vi "tower Controller.vi"(8 "error in":errorcluster) -> ()   [LabVIEW 2017]
doc: "This VI executes continuously carrying out the current operation and responding to updates or new operations. It will often contain the timing or control code that is difficult to place directly in TeleOp. This VI generally opens all sensors and motors and isolates the rest of the robot code from knowing how the operations are carried out."
uses:
  <vilib>/Rock Robotics/WPI/Framework/Completion Status.ctl
  tower Setpoints.ctl
  tower Operations.ctl
  <vilib>/Rock Robotics/SystemInterfaces/DIO/FPGA_DIOChannel.ctl
  <vilib>/Rock Robotics/WPI/Encoder/WPI_EncoderType.ctl
  <vilib>/Rock Robotics/SystemInterfaces/DIO/FPGA_DIOPWMChannel.ctl
  Public/Documents/Cross The Road Electronics/Phoenix-LabVIEW/Motor Controller/Controls/CTRE_Phoenix_MotorControl_ControlMode.ctl
  tower Published Globals.vi
  <vilib>/Rock Robotics/WPI/Counter/WPI_CounterDigitalInputToDigitalSource.vi
  Framework/Robot Global Data.vi
  <vilib>/Rock Robotics/Network Tables/NT Write Boolean.vi
panel:
  out "Arm Encoder":dbl
  out "TowerLastCommandStatus":T1=enum."Incomplete"
  in  "Interactive Values":T2
  out "Current\nCmd":string
  in  "Buttons":cluster{"Execute Cmd":bool, "Abort Cmd":bool}
  out "Command Timing":cluster{"Start Time (ms)":u32, "Iterations":i32}
  out "Status":T1
  # "Tip: It may be helpful to observe inputs and sensor values.\nYou may also want to display tuning or debugging controls.\nFor ArmPosition Setpoint is # of raw units to travel\nFor ArmReset Setpoint is motor speed (-1 to +1)\nDuration is #seconds to run (zero is reset is immediate).\n-Motor speed sp lowers arm, + motor speed sp raises arm.\nFor reset, motor will stop when limit swtich is made."
  # "Interactive Command: You may fill in the settings for a command\nand schedule it with the Execute button. You can observe and abort\nany command while fine tuning the code for the controller."
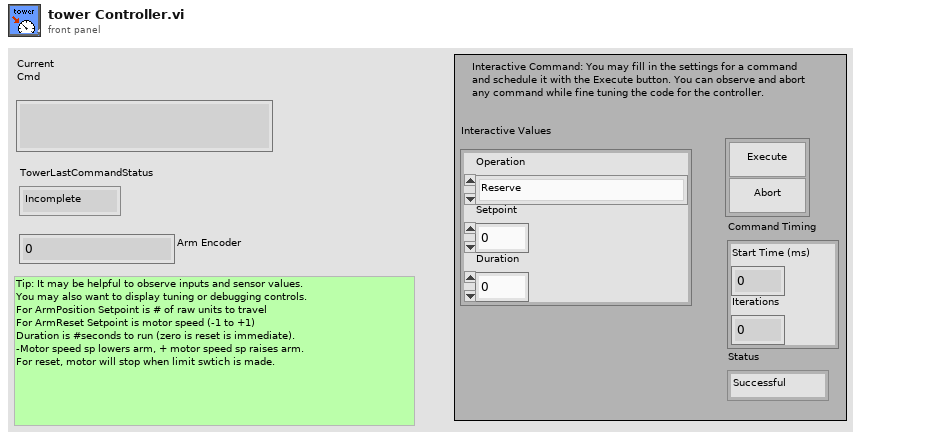
[diagram p1: front panel]
types:
  T1 = typedef "Completion Status.ctl" = enum16{"Successful", "Aborted", "Incomplete"}
  T2 = typedef "tower Setpoints.ctl" = cluster{"Operation":T3, "Setpoint":dbl, "Duration":dbl}
  T3 = typedef "tower Operations.ctl" = enum16{"Reserve", "Read Current", "Immediate", "LaunchClimber", "ArmReset", "ArmPosition", "TowerClimbImmediate"}
  T4 = typedef "FPGA_DIOPWMChannel.ctl" = enum8{"PWM 0", "PWM 1", "PWM 2", "PWM 3", "PWM 4", "PWM 5", "PWM 6", "PWM 7", "PWM 8", "PWM 9", "PWM MXP 0", "PWM MXP 1", "PWM MXP 2", "PWM MXP 3", "PWM MXP 4", "PWM MXP 5", "PWM MXP 6", "PWM MXP 7", "PWM MXP 8", "PWM MXP 9", "Invalid"}
  T5 = typedef "WPI_EncoderType.ctl" = enum16{"1x", "2x", "4x"}
  T6 = typedef "FPGA_DIOChannel.ctl" = enum8{"DIO 0", "DIO 1", "DIO 2", "DIO 3", "DIO 4", "DIO 5", "DIO 6", "DIO 7", "DIO 8", "DIO 9", "DIO MXP 0", "DIO MXP 1", "DIO MXP 2", "DIO MXP 3", "DIO MXP 4", "DIO MXP 5", "DIO MXP 6", "DIO MXP 7", "DIO MXP 8", "DIO MXP 9", "DIO MXP 10", "DIO MXP 11", "DIO MXP 12", "DIO MXP 13", "DIO MXP 14", "DIO MXP 15", "SPI Port CS1", "SPI Port CS2", "SPI Port CS3", "SPI Port MISO", "SPI Port MOSI", "Invalid"}
  T7 = typedef "WPI_DigitalOutputDevRef.ctl" = cluster{"DIO Channel":T6, "DevStatus":errorcluster}
  T8 = typedef "WPI_DigitalInputDevRef.ctl" = cluster{"DevStatus":errorcluster, "DIO Channel":T6}
  T9 = typedef "WPI_PWMDeviceRef.ctl" = cluster{"DeviceStatus":errorcluster, "PWM Channel":T4}
  T10 = typedef "FPGA_CounterEncoderSourceConvertionLVSourceType.ctl" = cluster{"DevStatus":errorcluster, "AnalogTriggerMode?":bool, "DigitalMode":cluster{"DIO Channel":T11}, "AnalogTriggerMode":cluster{"AnalogTriggerIndex":T12, "OutputType":T13}}
  T11 = typedef "FPGA_DIODigitalSourceChannel.ctl" = enum8{"DIO 0", "DIO 1", "DIO 2", "DIO 3", "DIO 4", "DIO 5", "DIO 6", "DIO 7", "DIO 8", "DIO 9", "DIO MXP 0", "DIO MXP 1", "DIO MXP 2", "DIO MXP 3", "DIO MXP 4", "DIO MXP 5", "DIO MXP 6", "DIO MXP 7", "DIO MXP 8", "DIO MXP 9", "DIO MXP 10", "DIO MXP 11", "DIO MXP 12", "DIO MXP 13", "DIO MXP 14", "DIO MXP 15", "Disabled"}
  T12 = typedef "FPGA_AnalogTriggerIndex.ctl" = enum8{"Trig 0", "Trig 1", "Trig 2", "Trig 3", "Trig 4", "Trig 5", "Trig 6", "Trig 7", "Invalid"}
  T13 = typedef "FPGA_AnalogTriggerOutType.ctl" = enum16{"InWindow", "TriggerState", "Rising", "Falling"}
  T14 = typedef "WPI_EncoderDevRef.ctl" = cluster{"DevStatus":errorcluster, "EncoderIndex":T15, "CounterIndex":T16, "DistancePerCount":dbl, "Decoding Type":T5}
  T15 = typedef "FPGA_EncoderIdx.ctl" = enum8{"Enc 0", "Enc 1", "Enc 2", "Enc 3", "Enc 4", "Enc 5", "Enc 6", "Enc 7", "Invalid"}
  T16 = typedef "FPGA_CounterCtrSystemIndex.ctl" = enum8{"Ctr 0", "Ctr 1", "Ctr 2", "Ctr 3", "Ctr 4", "Ctr 5", "Ctr 6", "Ctr 7", "Invalid"}
  T17 = typedef "WPI_MotorControlDeviceRef.ctl" = cluster{"DeviceStatus":errorcluster, "Type":T18, "PWM":cluster{"PWM Channel":T4, "DeadBand":T19}, "CAN":cluster{"Device Number":u8, "SetOutput VI Ref":variant, "GetOutput VI Ref":variant, "Enable VI Ref":variant, "Disable VI Ref":variant, "Data":variant}, "Invert":bool, "DIO PWM":cluster{"PWM \"Enable\" Channel":T4, "DIOChannel":T6, "PWM Rate":dbl}}
  T18 = typedef "WPI_MotorControlType.ctl" = enum16{"PWM", "CAN", "DIO PWM"}
  T19 = typedef "WPI_PWMDeadband.ctl" = cluster{"Name":string, "maxPositivePwm":i32, "minPositivePwm":i32, "centerPwm":i32, "maxNegativePwm":i32, "minNegativePwm":i32, "angularRange":u16}
  T20 = typedef "Command Status Info.ctl" = cluster{"Name":string, "Status":T1, "notifier out":T21}
  T21 = typedef "Completion Notifier.ctl" = refnum<notifier>
  T22 = cluster{"Current Command":T2, "Command Timing":cluster{"Start Time (ms)":u32, "Iterations":i32}, "Command Arguments":cluster{"Command Info":T20, "Description":string, "Default Command":T2, "queue out":refnum<queue>, "Subsystem Name":string}}
  T23 = typedef "CTRE_Phoenix_MotorControl_ControlMode.ctl" = u16
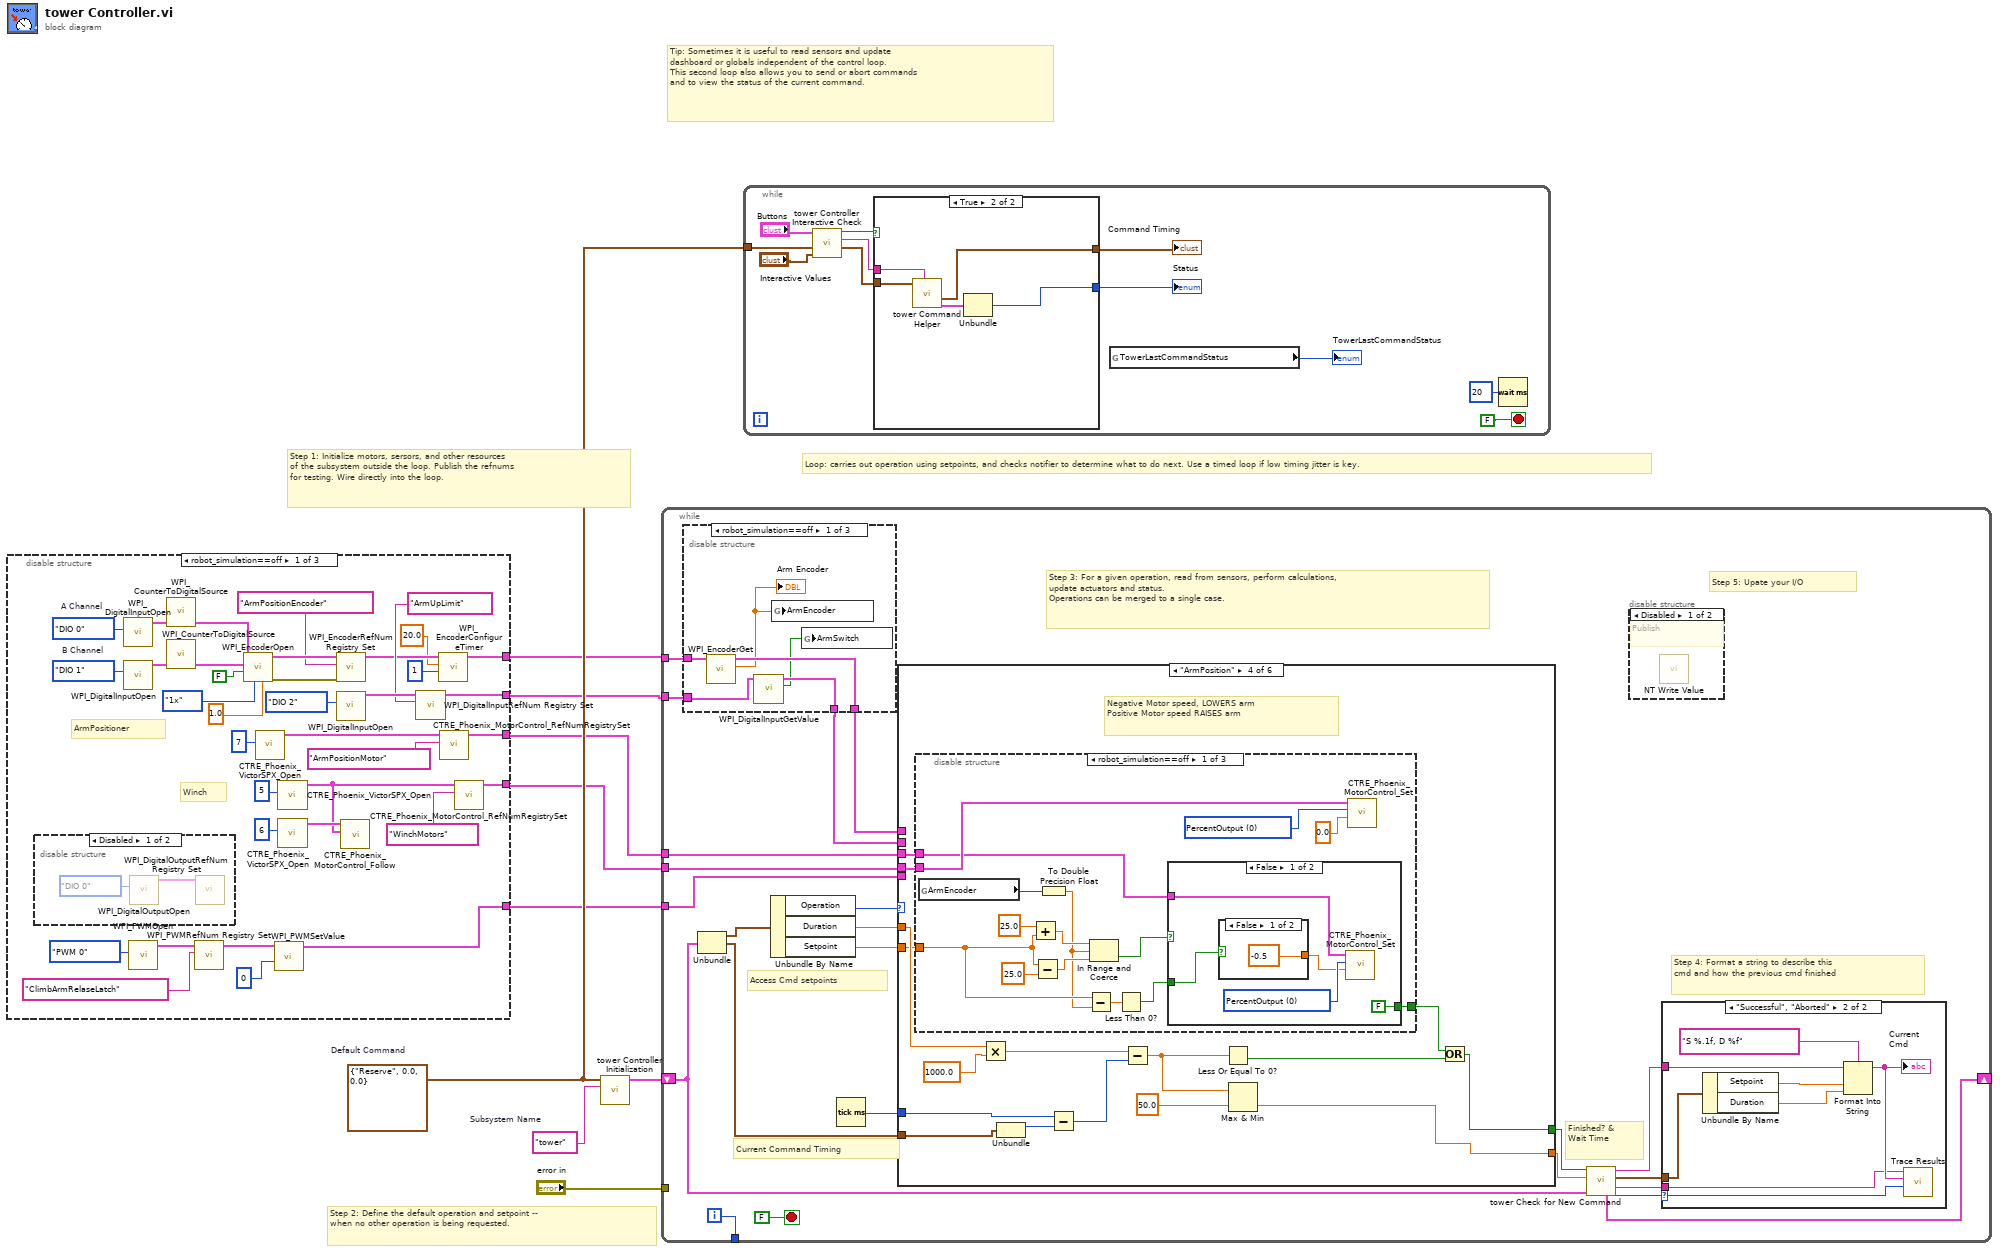
[diagram p0: block diagram]
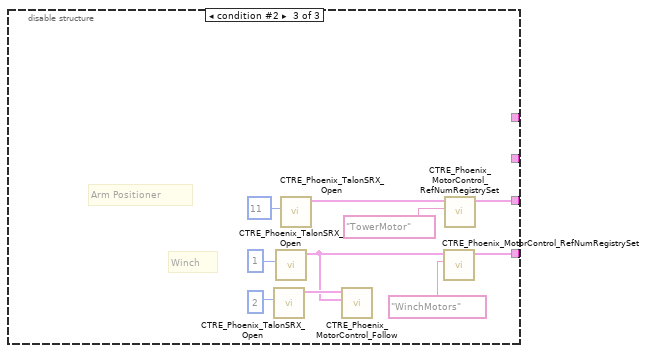
[diagram p4: hidden frame]
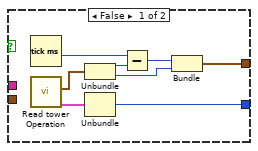
[diagram p5: hidden frame]
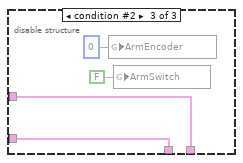
[diagram p7: hidden frame]
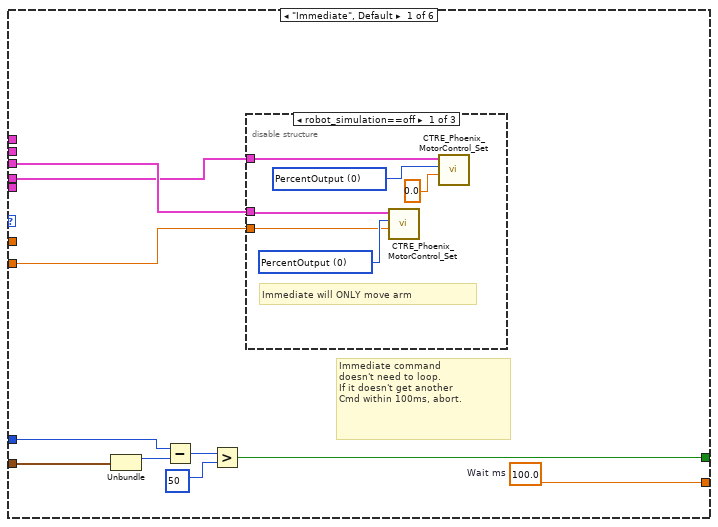
[diagram p10: hidden frame]
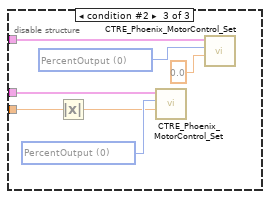
[diagram p12: hidden frame]
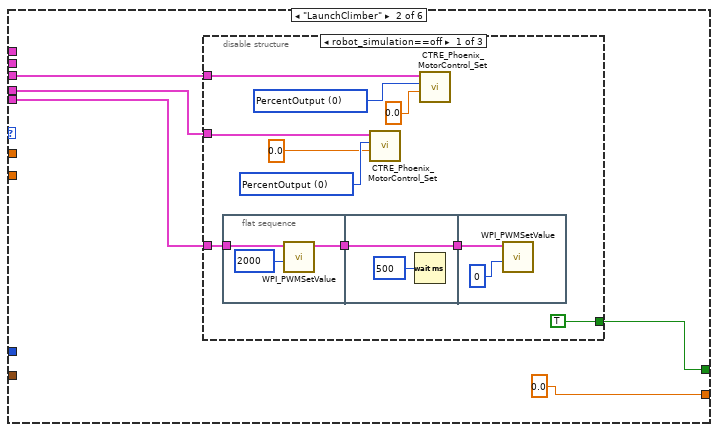
[diagram p13: hidden frame]
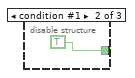
[diagram p14: hidden frame]
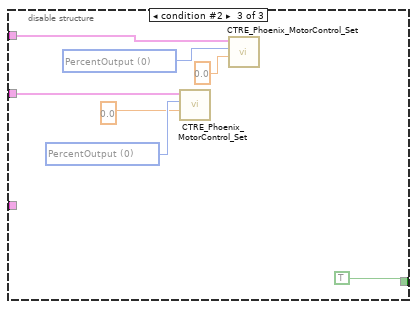
[diagram p15: hidden frame]
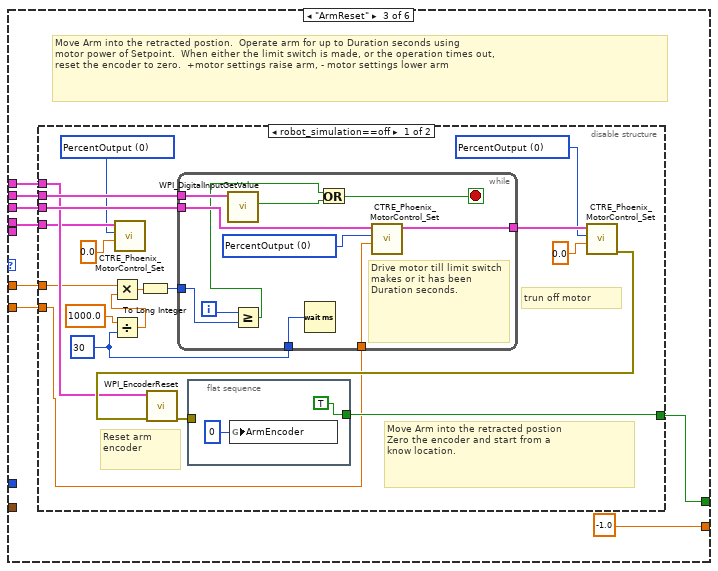
[diagram p16: hidden frame]
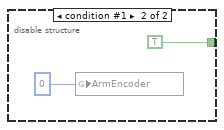
[diagram p17: hidden frame]
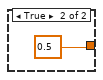
[diagram p18: hidden frame]
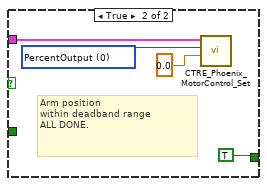
[diagram p19: hidden frame]
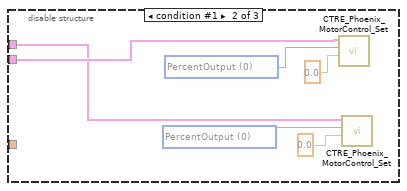
[diagram p20: hidden frame]
diagram:
  w6 = T2 {"Operation"=enum."Reserve", "Setpoint"=0.0, "Duration"=0.0}  # Default Command
  w7 = "tower"  # Subsystem Name
  # "Tip: Sometimes it is useful to read sensors and update\ndashboard or globals independent of the control loop.\nThis second loop also allows you to send or abort commands\nand to view the status of the current command."
  # "Step 2: Define the default operation and setpoint --\nwhen no other operation is being requested."
  # "Step 1: Initialize motors, sersors, and other resources\nof the subsystem outside the loop. Publish the refnums\nfor testing. Wire directly into the loop."
  # "Loop: carries out operation using setpoints, and checks notifier to determine what to do next. Use a timed loop if low timing jitter is key."
  n1 = disable-structure shown="robot_simulation==off" {
    disable-tunnel: [w37 _ w55] -> w5
    disable-tunnel: [w40 _ w51] -> w4
    disable-tunnel: [w22 _ _] -> w1
    disable-tunnel: [w24 _ _] -> w2
    disable-tunnel: [w13 _ _] -> w3
    frame condition #0 (active) {
      w35 = FPGA_DIOChannel."DIO 1"  # B Channel
      w34 = FPGA_DIOChannel."DIO 0"  # A Channel
      # "Winch"
      # "ArmPositioner"
      n2 = disable-structure shown="Disabled" {
        frame Disabled {
          n3 = call <vilib>:"WPI_DigitalOutputOpen.vi"("DIO Channel"=FPGA_DIOChannel."DIO 0") -> ("DigitalOutputDevRef"=w47:T7)  [unwired: 9 in, 1 out]
          n4 = call <vilib>:"WPI_DigitalOutputRefNum Registry Set.vi"("DigitalOutputDevRef"=w47) -> ()  [unwired: 9 in, 2 out]
        }
        frame Enabled {
        }
      }
      n5 = call <vilib>:"WPI_DigitalInputOpen.vi"("DIO Channel"=w34) -> ("DigitalInputDevRef"=w31:T8)  [unwired: 1 in, 9 out]
      n6 = call <vilib>:"WPI_DigitalInputOpen.vi"("DIO Channel"=w35) -> ("DigitalInputDevRef"=w32:T8)  [unwired: 1 in, 9 out]
      n7 = call <vilib>:"WPI_PWMOpen.vi"("PWM Channel"=FPGA_DIOPWMChannel."PWM 0") -> ("PWMDeviceRef"=w16:T9)  [unwired: 9 in, 1 out]
      n8 = call-poly <vilib>:"WPI_CounterToDigitalSource.vi"("DigitalInputDevRef"=w31) -> ("Digital Source"=w30:T10)  [unwired: 6 out]
      n9 = call-poly <vilib>:"WPI_CounterToDigitalSource.vi"("DigitalInputDevRef"=w32) -> ("Digital Source"=w33:T10)  [unwired: 6 out]
      n10 = call <vilib>:"WPI_PWMRefNum Registry Set.vi"("refnum name"="ClimbArmRelaseLatch", "PWMDeviceRef"=w16) -> ("PWMDeviceRef"=w15:T9)  [unwired: 8 in, 1 out]
      n11 = call <vilib>:"WPI_EncoderOpen.vi"("DistancePerCount"=1.0, "Decoding Type"=WPI_EncoderType."1x", "Invert Direction (False)"=FALSE, "BSource"=w33, "ASource"=w30) -> ("error out"=w29:errorcluster, "EncoderDevRef"=w28:T14)  [unwired: 3 in, 2 out]
      n12 = call "CTRE_Phoenix_VictorSPX_Open.vi"("Device Number"=u8 7) -> ("CAN Talon SRX Ref"=w38:T17)  [unwired: 9 in, 1 out]
      n13 = call <vilib>:"WPI_PWMSetValue.vi"("Value"=u16 0, "PWMDeviceRef"=w15) -> ("PWMDeviceRef"=w13:T9)  [unwired: 8 in, 1 out]
      n14 = call "CTRE_Phoenix_VictorSPX_Open.vi"("Device Number"=u8 5) -> ("CAN Talon SRX Ref"=w41:T17)  [unwired: 9 in, 1 out]
      n15 = call "CTRE_Phoenix_VictorSPX_Open.vi"("Device Number"=u8 6) -> ("CAN Talon SRX Ref"=w42:T17)  [unwired: 9 in, 1 out]
      n16 = call <vilib>:"WPI_EncoderRefNum Registry Set.vi"("error in (no error)"=w29, "refnum name"="ArmPositionEncoder", "EncoderDevRef"=w28) -> ("EncoderDevRef"=w21:T14)  [unwired: 7 in, 1 out]
      n17 = call <vilib>:"WPI_DigitalInputOpen.vi"("DIO Channel"=FPGA_DIOChannel."DIO 2") -> ("DigitalInputDevRef"=w25:T8)  [unwired: 9 in, 1 out]
      n18 = call "CTRE_Phoenix_MotorControl_Follow.vi"("Master Controller to Follow"=w41, "PhoenixMotorControlDevRef"=w42) -> ()  [unwired: 8 in, 2 out]
      n19 = call <vilib>:"WPI_DigitalInputRefNum Registry Set.vi"("refnum name"="ArmUpLimit", "DigitalInputDevRef"=w25) -> ("DigitalInputDevRef"=w24:T8)  [unwired: 8 in, 1 out]
      n20 = call <vilib>:"WPI_EncoderConfigureTimer.vi"("Number Samples to Average"=u8 1, "Minimum Rate"=20.0, "EncoderDevRef"=w21) -> ("EncoderDevRef"=w22:T14)  [unwired: 7 in, 1 out]
      n21 = call "CTRE_Phoenix_MotorControl_RefNumRegistrySet.vi"("refnum name"="ArmPositionMotor", "PhoenixMotorControlDevRef"=w38) -> ("PhoenixMotorControlDevRef"=w37:T17)  [unwired: 8 in, 1 out]
      n22 = call "CTRE_Phoenix_MotorControl_RefNumRegistrySet.vi"("refnum name"="WinchMotors", "PhoenixMotorControlDevRef"=w41) -> ("PhoenixMotorControlDevRef"=w40:T17)  [unwired: 8 in, 1 out]
    }
    frame condition #1 {
    }
    frame condition #2 {
      # "Winch"
      # "Arm Positioner"
      n23 = call "CTRE_Phoenix_TalonSRX_Open.vi"("Device Number"=u8 2) -> ("CAN Talon SRX Ref"=w49:T17)  [unwired: 9 in, 1 out]
      n24 = call "CTRE_Phoenix_TalonSRX_Open.vi"("Device Number"=u8 1) -> ("CAN Talon SRX Ref"=w48:T17)  [unwired: 9 in, 1 out]
      n25 = call "CTRE_Phoenix_TalonSRX_Open.vi"("Device Number"=u8 11) -> ("CAN Talon SRX Ref"=w56:T17)  [unwired: 9 in, 1 out]
      n26 = call "CTRE_Phoenix_MotorControl_Follow.vi"("Master Controller to Follow"=w48, "PhoenixMotorControlDevRef"=w49) -> ()  [unwired: 8 in, 2 out]
      n27 = call "CTRE_Phoenix_MotorControl_RefNumRegistrySet.vi"("refnum name"="WinchMotors", "PhoenixMotorControlDevRef"=w48) -> ("PhoenixMotorControlDevRef"=w51:T17)  [unwired: 8 in, 1 out]
      n28 = call "CTRE_Phoenix_MotorControl_RefNumRegistrySet.vi"("refnum name"="TowerMotor", "PhoenixMotorControlDevRef"=w56) -> ("PhoenixMotorControlDevRef"=w55:T17)  [unwired: 8 in, 1 out]
    }
  }
  n29 = call "tower Controller Initialization.vi"("Subsystem Name"=w7, "Default Command"=w6) -> ("Current Command"=w8:T22)  [unwired: 9 in]
  n30 = while {
    shift-right: [w72] -> _
    shift-left: w8 -> [w67]
    tunnel: [w79] -> _
    tunnel: "error in" -> [_]
    tunnel: w5 -> [w66]
    tunnel: w4 -> [w65]
    tunnel: w1 -> [w58]
    tunnel: w2 -> [w62]
    tunnel: w3 -> [w61]
    i -> [w79]
    stop <- FALSE stop-if-true
    # "Step 5: Upate your I/O"
    # "Step 4: Format a string to describe this\ncmd and how the previous cmd finished"
    # "Current Command Timing"
    # "Access Cmd setpoints"
    # "Finished? &\nWait Time"
    # "Step 3: For a given operation, read from sensors, perform calculations,\nupdate actuators and status.\nOperations can be merged to a single case."
    n31 = disable-structure shown="robot_simulation==off" {
      disable-tunnel: w58 -> [w82 w88 w91]
      disable-tunnel: [w86 w88 w91] -> w64
      disable-tunnel: w62 -> [w85 w87 w90]
      disable-tunnel: [w84 w87 w90] -> w63
      frame condition #0 (active) {
        n32 = call <vilib>:"WPI_EncoderGet.vi"("EncoderDevRef"=w82) -> ("Distance"=w81:dbl, "EncoderDevRef"=w86:T14)  [unwired: 5 in, 4 out]
        "Arm Encoder" <- w81
        n33 = call <vilib>:"WPI_DigitalInputGetValue.vi"("DigitalInputDevRef"=w85) -> ("Value"=w83:bool, "DigitalInputDevRef"=w84:T8)  [unwired: 8 in, 1 out]
        n34 = global write "Robot Global Data.vi" "ArmEncoder"(w81) -> ()
        n35 = global write "Robot Global Data.vi" "ArmSwitch"(w83) -> ()
      }
      frame condition #1 {
      }
      frame condition #2 {
        n36 = global write "Robot Global Data.vi" "ArmEncoder"(0 ("ArmEncoder")) -> ()
        n37 = global write "Robot Global Data.vi" "ArmSwitch"(FALSE ("ArmSwitch")) -> ()
      }
    }
    n38 = Unbundle(w67) -> ("Current Command"=w78:T2, "Command Timing"=w74:cluster{"Start Time (ms)":u32, "Iterations":i32})  [unwired: 1 out]
    n39 = Unbundle By Name(w78) -> ("Operation"=w77:T3, "Duration"=w76:dbl, "Setpoint"=w73:dbl)
    n40 = Tick Count (ms)() -> (millisecond timer value=w75:u32)
    n41 = case shown="\"ArmPosition\"" w77 {
      tunnel: [w110 0.0 ("Infinite") -1.0 ("Infinite") w204 100.0 w262] -> w59
      tunnel: [w104 w124 w157 w201 FALSE ("ignore previous (F)") w263] -> w60
      tunnel: w74 -> [w106 _ _ w206 _ w265]
      tunnel: w76 -> [_ _ w155 w203 _ _]
      tunnel: w75 -> [w105 _ _ w205 _ w264]
      tunnel: w73 -> [w102 _ w154 w198 _ w261]
      tunnel: w66 -> [w103 w126 w159 w197 w246 w259]
      tunnel: w65 -> [w101 w127 w156 w202 w245 w260]
      tunnel: w64 -> [_ _ w158 _ _ _]
      tunnel: w63 -> [_ _ w160 _ _ _]
      tunnel: w61 -> [_ w125 _ _ _ _]
      frame "Immediate", Default {
        w110 = 100.0  # Wait ms
        # "Immediate command\ndoesn't need to loop.\nIf it doesn't get another\nCmd within 100ms, abort."
        n42 = Unbundle(w106) -> ("Start Time (ms)"=w109:u32)  [unwired: 1 out]
        n43 = Subtract(x=w105, y=w109) -> (x-y=w108:u32)
        n44 = Greater?(x=w108, y=u8 50 ("Left Motor")) -> (0:w104:bool)
        n45 = disable-structure shown="robot_simulation==off" {
          disable-tunnel: w103 -> [w116 _ w123]
          disable-tunnel: w102 -> [w111 _ w121]
          disable-tunnel: w101 -> [w112 _ w117]
          frame condition #0 (active) {
            w113 = T23 0 items=["PercentOutput"=0, "Position"=1, "Velocity"=2, "Current"=3, "Follower"=5, "MotionProfile"=6, "MotionMagic"=7, "MotionMagicArc"=8, "MotionProfileArc"=10, "Disabled"=15] ("Control Mode")
            w115 = T23 0 items=["PercentOutput"=0, "Position"=1, "Velocity"=2, "Current"=3, "Follower"=5, "MotionProfile"=6, "MotionMagic"=7, "MotionMagicArc"=8, "MotionProfileArc"=10, "Disabled"=15] ("Control Mode")
            # "Immediate will ONLY move arm"
            n46 = call "CTRE_Phoenix_MotorControl_Set.vi"("Output"=w111, "Control Mode"=w115, "PhoenixMotorControlDevRef"=w116) -> ()  [unwired: 7 in, 2 out]
            n47 = call "CTRE_Phoenix_MotorControl_Set.vi"("Output"=0.0, "Control Mode"=w113, "PhoenixMotorControlDevRef"=w112) -> ()  [unwired: 7 in, 2 out]
          }
          frame condition #1 {
          }
          frame condition #2 {
            w118 = T23 0 items=["PercentOutput"=0, "Position"=1, "Velocity"=2, "Current"=3, "Follower"=5, "MotionProfile"=6, "MotionMagic"=7, "MotionMagicArc"=8, "MotionProfileArc"=10, "Disabled"=15] ("Control Mode")
            w122 = T23 0 items=["PercentOutput"=0, "Position"=1, "Velocity"=2, "Current"=3, "Follower"=5, "MotionProfile"=6, "MotionMagic"=7, "MotionMagicArc"=8, "MotionProfileArc"=10, "Disabled"=15] ("Control Mode")
            n48 = Absolute Value(x=w121) -> (abs(x)=w120:dbl)
            n49 = call "CTRE_Phoenix_MotorControl_Set.vi"("Output"=w120, "Control Mode"=w122, "PhoenixMotorControlDevRef"=w123) -> ()  [unwired: 7 in, 2 out]
            n50 = call "CTRE_Phoenix_MotorControl_Set.vi"("Output"=0.0, "Control Mode"=w118, "PhoenixMotorControlDevRef"=w117) -> ()  [unwired: 7 in, 2 out]
          }
        }
      }
      frame "LaunchClimber" {
        n51 = disable-structure shown="robot_simulation==off" {
          disable-tunnel: w127 -> [w133 _ w153]
          disable-tunnel: w126 -> [w134 _ w149]
          disable-tunnel: w125 -> [w132 _ _]
          disable-tunnel: [TRUE ("ignore previous (F)") TRUE ("ignore previous (F)") TRUE ("ignore previous (F)")] -> w124
          frame condition #0 (active) {
            w136 = T23 0 items=["PercentOutput"=0, "Position"=1, "Velocity"=2, "Current"=3, "Follower"=5, "MotionProfile"=6, "MotionMagic"=7, "MotionMagicArc"=8, "MotionProfileArc"=10, "Disabled"=15] ("Control Mode")
            w138 = T23 0 items=["PercentOutput"=0, "Position"=1, "Velocity"=2, "Current"=3, "Follower"=5, "MotionProfile"=6, "MotionMagic"=7, "MotionMagicArc"=8, "MotionProfileArc"=10, "Disabled"=15] ("Control Mode")
            n52 = flat-sequence {
              tunnel: w132 -> [w140]
              tunnel: [w141] -> w130
              tunnel: [w142] -> w131
              tunnel: w130 -> [w142]
              tunnel: w131 -> [w145]
              frame #0 {
                n53 = call <vilib>:"WPI_PWMSetValue.vi"("Value"=u16 2000, "PWMDeviceRef"=w140) -> ("PWMDeviceRef"=w141:T9)  [unwired: 8 in, 1 out]
              }
              frame #1 {
                n54 = Wait (ms)(milliseconds to wait=u32 500) -> ()  [unwired: 1 out]
              }
              frame #2 {
                n55 = call <vilib>:"WPI_PWMSetValue.vi"("Value"=u16 0, "PWMDeviceRef"=w145) -> ()  [unwired: 8 in, 2 out]
              }
            }
            n56 = call "CTRE_Phoenix_MotorControl_Set.vi"("Output"=0.0, "Control Mode"=w138, "PhoenixMotorControlDevRef"=w133) -> ()  [unwired: 7 in, 2 out]
            n57 = call "CTRE_Phoenix_MotorControl_Set.vi"("Output"=0.0, "Control Mode"=w136, "PhoenixMotorControlDevRef"=w134) -> ()  [unwired: 7 in, 2 out]
          }
          frame condition #1 {
          }
          frame condition #2 {
            w150 = T23 0 items=["PercentOutput"=0, "Position"=1, "Velocity"=2, "Current"=3, "Follower"=5, "MotionProfile"=6, "MotionMagic"=7, "MotionMagicArc"=8, "MotionProfileArc"=10, "Disabled"=15] ("Control Mode")
            w152 = T23 0 items=["PercentOutput"=0, "Position"=1, "Velocity"=2, "Current"=3, "Follower"=5, "MotionProfile"=6, "MotionMagic"=7, "MotionMagicArc"=8, "MotionProfileArc"=10, "Disabled"=15] ("Control Mode")
            n58 = call "CTRE_Phoenix_MotorControl_Set.vi"("Output"=0.0, "Control Mode"=w152, "PhoenixMotorControlDevRef"=w153) -> ()  [unwired: 7 in, 2 out]
            n59 = call "CTRE_Phoenix_MotorControl_Set.vi"("Output"=0.0, "Control Mode"=w150, "PhoenixMotorControlDevRef"=w149) -> ()  [unwired: 7 in, 2 out]
          }
        }
      }
      frame "ArmReset" {
        # "Move Arm into the retracted postion.  Operate arm for up to Duration seconds using\nmotor power of Setpoint.  When either the limit switch is made, or the operation times out,\nreset the encoder to zero.  +motor settings raise arm, - motor settings lower arm"
        n60 = disable-structure shown="robot_simulation==off" {
          disable-tunnel: w160 -> [w180 _]
          disable-tunnel: w159 -> [w179 _]
          disable-tunnel: w158 -> [w174 _]
          disable-tunnel: [w172 TRUE] -> w157
          disable-tunnel: w156 -> [w171 _]
          disable-tunnel: w155 -> [w168 _]
          disable-tunnel: w154 -> [w162 _]
          frame condition #0 (active) {
            w163 = u32 30 ("milliseconds to wait")
            w169 = T23 0 items=["PercentOutput"=0, "Position"=1, "Velocity"=2, "Current"=3, "Follower"=5, "MotionProfile"=6, "MotionMagic"=7, "MotionMagicArc"=8, "MotionProfileArc"=10, "Disabled"=15] ("Control Mode")
            w177 = T23 0 items=["PercentOutput"=0, "Position"=1, "Velocity"=2, "Current"=3, "Follower"=5, "MotionProfile"=6, "MotionMagic"=7, "MotionMagicArc"=8, "MotionProfileArc"=10, "Disabled"=15] ("Control Mode")
            # "Reset arm \nencoder"
            # "trun off motor"
            # "Move Arm into the retracted postion\nZero the encoder and start from a \nknow location."
            n61 = Divide(x=1000.0 ("y"), y=w163) -> (x/y=w166:dbl)
            n62 = Multiply(x=w168, y=w166) -> (x*y=w165:dbl)
            n63 = call "CTRE_Phoenix_MotorControl_Set.vi"("Output"=0.0, "Control Mode"=w169, "PhoenixMotorControlDevRef"=w171) -> ()  [unwired: 7 in, 2 out]
            n64 = To Long Integer(number=w165) -> (32bit integer=w164:i32)
            n65 = while {
              tunnel: w180 -> [w193]
              tunnel: w179 -> [w192]
              tunnel: [w190] -> w178
              tunnel: w164 -> [w183]
              tunnel: w163 -> [w186]
              tunnel: w162 -> [w185]
              i -> [w184]
              stop <- w187 stop-if-true
              w191 = T23 0 items=["PercentOutput"=0, "Position"=1, "Velocity"=2, "Current"=3, "Follower"=5, "MotionProfile"=6, "MotionMagic"=7, "MotionMagicArc"=8, "MotionProfileArc"=10, "Disabled"=15] ("Control Mode")
              # "Drive motor till limit switch makes or it has been Duration seconds."
              n66 = call <vilib>:"WPI_DigitalInputGetValue.vi"("DigitalInputDevRef"=w193) -> ("Value"=w188:bool)  [unwired: 8 in, 2 out]
              n67 = Greater Or Equal?(x=w184, y=w183) -> (x >= y?=w189:bool)
              n68 = Wait (ms)(milliseconds to wait=w186) -> ()  [unwired: 1 out]
              n69 = Or(x=w189, y=w188) -> (x .or. y?=w187:bool)
              n70 = call "CTRE_Phoenix_MotorControl_Set.vi"("Output"=w185, "Control Mode"=w191, "PhoenixMotorControlDevRef"=w192) -> ("PhoenixMotorControlDevRef"=w190:T17)  [unwired: 7 in, 1 out]
            }
            n71 = flat-sequence {
              tunnel: w173 -> [_]
              tunnel: [TRUE] -> w172
              frame #0 {
                n72 = global write "Robot Global Data.vi" "ArmEncoder"(0 ("ArmEncoder")) -> ()
              }
            }
            n73 = call "CTRE_Phoenix_MotorControl_Set.vi"("Output"=0.0, "Control Mode"=w177, "PhoenixMotorControlDevRef"=w178) -> ("error out"=w175:errorcluster)  [unwired: 7 in, 1 out]
            n74 = call <vilib>:"WPI_EncoderReset.vi"("error in (no error)"=w175, "EncoderDevRef"=w174) -> ("error out"=w173:errorcluster)  [unwired: 8 in, 1 out]
          }
          frame condition #1 {
            n75 = global write "Robot Global Data.vi" "ArmEncoder"(0 ("ArmEncoder")) -> ()
          }
        }
      }
      frame "ArmPosition" {
        # "Negative Motor speed, LOWERS arm\nPositive Motor speed RAISES arm"
        n76 = disable-structure shown="robot_simulation==off" {
          disable-tunnel: w202 -> [w226 w239 _]
          disable-tunnel: [w219 _ _] -> w199
          disable-tunnel: w198 -> [w218 _ _]
          disable-tunnel: w197 -> [w214 w238 _]
          frame condition #0 (active) {
            w212 = T23 0 items=["PercentOutput"=0, "Position"=1, "Velocity"=2, "Current"=3, "Follower"=5, "MotionProfile"=6, "MotionMagic"=7, "MotionMagicArc"=8, "MotionProfileArc"=10, "Disabled"=15] ("Control Mode")
            n77 = global read "Robot Global Data.vi" "ArmEncoder"() -> (w221:i32)
            n78 = Add(x=25.0, y=w218) -> (x+y=w225:dbl)
            n79 = Subtract(x=w218, y=25.0 ("x")) -> (x-y=w222:dbl)
            n80 = To Double Precision Float(number=w221) -> (double precision float=w217:dbl)
            n81 = Subtract(x=w218, y=w217) -> (x-y=w216:dbl)
            n82 = In Range and Coerce(upper limit=w225, x=w217, lower limit=w222) -> (In Range?=w220:bool)  [unwired: 1 out]
            n83 = Less Than 0?(x=w216) -> (x < 0?=w215:bool)
            n84 = case shown="False" w220 {
              tunnel: [FALSE TRUE] -> w219
              tunnel: w215 -> [w229 _]
              tunnel: w214 -> [w227 w236]
              frame False {
                w230 = T23 0 items=["PercentOutput"=0, "Position"=1, "Velocity"=2, "Current"=3, "Follower"=5, "MotionProfile"=6, "MotionMagic"=7, "MotionMagicArc"=8, "MotionProfileArc"=10, "Disabled"=15] ("Control Mode")
                n85 = case shown="False" w229 {
                  tunnel: [-0.5 ("Output") 0.5 ("Output")] -> w228
                  frame False {
                  }
                  frame True {
                  }
                }
                n86 = call "CTRE_Phoenix_MotorControl_Set.vi"("Output"=w228, "Control Mode"=w230, "PhoenixMotorControlDevRef"=w227) -> ()  [unwired: 7 in, 2 out]
              }
              frame True {
                w235 = T23 0 items=["PercentOutput"=0, "Position"=1, "Velocity"=2, "Current"=3, "Follower"=5, "MotionProfile"=6, "MotionMagic"=7, "MotionMagicArc"=8, "MotionProfileArc"=10, "Disabled"=15] ("Control Mode")
                # "Arm position\nwithin deadband range\nALL DONE."
                n87 = call "CTRE_Phoenix_MotorControl_Set.vi"("Output"=0.0, "Control Mode"=w235, "PhoenixMotorControlDevRef"=w236) -> ()  [unwired: 7 in, 2 out]
              }
            }
            n88 = call "CTRE_Phoenix_MotorControl_Set.vi"("Output"=0.0, "Control Mode"=w212, "PhoenixMotorControlDevRef"=w226) -> ()  [unwired: 7 in, 2 out]
          }
          frame condition #1 {
            w241 = T23 0 items=["PercentOutput"=0, "Position"=1, "Velocity"=2, "Current"=3, "Follower"=5, "MotionProfile"=6, "MotionMagic"=7, "MotionMagicArc"=8, "MotionProfileArc"=10, "Disabled"=15] ("Control Mode")
            w242 = T23 0 items=["PercentOutput"=0, "Position"=1, "Velocity"=2, "Current"=3, "Follower"=5, "MotionProfile"=6, "MotionMagic"=7, "MotionMagicArc"=8, "MotionProfileArc"=10, "Disabled"=15] ("Control Mode")
            n89 = call "CTRE_Phoenix_MotorControl_Set.vi"("Output"=0.0, "Control Mode"=w242, "PhoenixMotorControlDevRef"=w239) -> ()  [unwired: 7 in, 2 out]
            n90 = call "CTRE_Phoenix_MotorControl_Set.vi"("Output"=0.0, "Control Mode"=w241, "PhoenixMotorControlDevRef"=w238) -> ()  [unwired: 7 in, 2 out]
          }
          frame condition #2 {
          }
        }
        n91 = Multiply(x=w203, y=1000.0) -> (x*y=w210:dbl)
        n92 = Unbundle(w206) -> ("Start Time (ms)"=w209:u32)  [unwired: 1 out]
        n93 = Subtract(x=w205, y=w209) -> (x-y=w211:u32)
        n94 = Subtract(x=w210, y=w211) -> (x-y=w208:dbl)
        n95 = Less Or Equal To 0?(x=w208) -> (x <= 0?=w200:bool)
        n96 = Max & Min(x=w208, y=50.0) -> (min(x,y)=w204:dbl)  [unwired: 1 out]
        n97 = Or(x=w199, y=w200) -> (x .or. y?=w201:bool)
      }
      frame "Reserve" {
        # "Encoder needs to be polled,\nuse 100ms wait for command\nbefore checking sensors"
        # "If loop needs to poll sensors or other\nvalues, use a timeout value. -1 waits for\nnext command to be sent."
        n98 = disable-structure shown="robot_simulation==off" {
          disable-tunnel: w246 -> [w252 _ w257]
          disable-tunnel: w245 -> [w251 _ w255]
          disable-tunnel: 0.0 ("Output") -> [w249 _ w254]
          frame condition #0 (active) {
            w250 = T23 0 items=["PercentOutput"=0, "Position"=1, "Velocity"=2, "Current"=3, "Follower"=5, "MotionProfile"=6, "MotionMagic"=7, "MotionMagicArc"=8, "MotionProfileArc"=10, "Disabled"=15] ("Control Mode")
            w253 = T23 0 items=["PercentOutput"=0, "Position"=1, "Velocity"=2, "Current"=3, "Follower"=5, "MotionProfile"=6, "MotionMagic"=7, "MotionMagicArc"=8, "MotionProfileArc"=10, "Disabled"=15] ("Control Mode")
            n99 = call "CTRE_Phoenix_MotorControl_Set.vi"("Output"=w249, "Control Mode"=w253, "PhoenixMotorControlDevRef"=w251) -> ()  [unwired: 7 in, 2 out]
            n100 = call "CTRE_Phoenix_MotorControl_Set.vi"("Output"=w249, "Control Mode"=w250, "PhoenixMotorControlDevRef"=w252) -> ()  [unwired: 7 in, 2 out]
          }
          frame condition #1 {
          }
          frame condition #2 {
            w256 = T23 0 items=["PercentOutput"=0, "Position"=1, "Velocity"=2, "Current"=3, "Follower"=5, "MotionProfile"=6, "MotionMagic"=7, "MotionMagicArc"=8, "MotionProfileArc"=10, "Disabled"=15] ("Control Mode")
            w258 = T23 0 items=["PercentOutput"=0, "Position"=1, "Velocity"=2, "Current"=3, "Follower"=5, "MotionProfile"=6, "MotionMagic"=7, "MotionMagicArc"=8, "MotionProfileArc"=10, "Disabled"=15] ("Control Mode")
            n101 = call "CTRE_Phoenix_MotorControl_Set.vi"("Output"=w254, "Control Mode"=w258, "PhoenixMotorControlDevRef"=w257) -> ()  [unwired: 7 in, 2 out]
            n102 = call "CTRE_Phoenix_MotorControl_Set.vi"("Output"=w254, "Control Mode"=w256, "PhoenixMotorControlDevRef"=w255) -> ()  [unwired: 7 in, 2 out]
          }
        }
      }
      frame "TowerClimbImmediate" {
        w262 = 100.0  # Wait ms
        # "Immediate command\ndoesn't need to loop.\nIf it doesn't get another\nCmd within 100ms, abort."
        n103 = Unbundle(w265) -> ("Start Time (ms)"=w268:u32)  [unwired: 1 out]
        n104 = Subtract(x=w264, y=w268) -> (x-y=w267:u32)
        n105 = Greater?(x=w267, y=u8 50 ("Left Motor")) -> (0:w263:bool)
        n106 = disable-structure shown="robot_simulation==off" {
          disable-tunnel: w260 -> [w273 _ w280]
          disable-tunnel: w261 -> [w272 _ w278]
          disable-tunnel: w259 -> [w269 _ w275]
          frame condition #0 (active) {
            w271 = T23 0 items=["PercentOutput"=0, "Position"=1, "Velocity"=2, "Current"=3, "Follower"=5, "MotionProfile"=6, "MotionMagic"=7, "MotionMagicArc"=8, "MotionProfileArc"=10, "Disabled"=15] ("Control Mode")
            w274 = T23 0 items=["PercentOutput"=0, "Position"=1, "Velocity"=2, "Current"=3, "Follower"=5, "MotionProfile"=6, "MotionMagic"=7, "MotionMagicArc"=8, "MotionProfileArc"=10, "Disabled"=15] ("Control Mode")
            # "ClimgImmediate will ONLY move winch"
            n107 = call "CTRE_Phoenix_MotorControl_Set.vi"("Output"=w272, "Control Mode"=w274, "PhoenixMotorControlDevRef"=w273) -> ()  [unwired: 7 in, 2 out]
            n108 = call "CTRE_Phoenix_MotorControl_Set.vi"("Output"=0.0, "Control Mode"=w271, "PhoenixMotorControlDevRef"=w269) -> ()  [unwired: 7 in, 2 out]
          }
          frame condition #1 {
          }
          frame condition #2 {
            w277 = T23 0 items=["PercentOutput"=0, "Position"=1, "Velocity"=2, "Current"=3, "Follower"=5, "MotionProfile"=6, "MotionMagic"=7, "MotionMagicArc"=8, "MotionProfileArc"=10, "Disabled"=15] ("Control Mode")
            w279 = T23 0 items=["PercentOutput"=0, "Position"=1, "Velocity"=2, "Current"=3, "Follower"=5, "MotionProfile"=6, "MotionMagic"=7, "MotionMagicArc"=8, "MotionProfileArc"=10, "Disabled"=15] ("Control Mode")
            n109 = call "CTRE_Phoenix_MotorControl_Set.vi"("Output"=w278, "Control Mode"=w279, "PhoenixMotorControlDevRef"=w280) -> ()  [unwired: 7 in, 2 out]
            n110 = call "CTRE_Phoenix_MotorControl_Set.vi"("Output"=0.0, "Control Mode"=w277, "PhoenixMotorControlDevRef"=w275) -> ()  [unwired: 7 in, 2 out]
          }
        }
      }
    }
    n111 = call "tower Check for New Command.vi"("Current Command"=w67, "Wait time (ms)"=w59, "Finished?"=w60) -> ("Completion"=w68:T1, "Subsystem Name"=w69:string, "Current Command"=w70:T2, "Initial Trace String"=w71:string, "NextCommand"=w72:T22)  [unwired: 4 in]
    n112 = disable-structure shown="Disabled" {
      frame Disabled {
        # "Publish"
        n113 = call-poly <vilib>:"NT Write Value.vi"() -> ()  [unwired: 11 in, 1 out]
      }
      frame Enabled {
      }
    }
    n114 = case shown="\"Successful\", \"Aborted\"" w68 {
      selector: w68 -> [_ w100]
      tunnel: w71 -> [_ w96]
      tunnel: w70 -> [_ w97]
      tunnel: w69 -> [_ w93]
      frame "Incomplete", Default {
        # "Continuing current command"
      }
      frame "Successful", "Aborted" {
        # "Report and setup for next command"
        n115 = Unbundle By Name(w97) -> ("Setpoint"=w99:dbl, "Duration"=w94:dbl)
        n116 = Format Into String(format string="S %.1f, D %f", initial string=w96, w99, w94) -> (resulting string=w95:string)  [unwired: 1 in, 1 out]
        "Current\nCmd" <- w95
        n117 = call <vilib>:"Trace Results.vi"("Status of previous command"=w100, "Description"=w95, "Subsystem"=w93) -> ()  [unwired: 9 in]
      }
    }
  }
  n118 = while {
    tunnel: w6 -> [w288]
    stop <- FALSE stop-if-true
    n119 = call "tower Controller Interactive Check.vi"("Interactive Command in"="Interactive Values", "Default Command"=w288, "Buttons"="Buttons") -> ("Interactive Command out"=w285:T2, "Trace String"=w286:string, "Schedule"=w287:bool)  [unwired: 6 in]
    n120 = case shown="True" w287 {
      tunnel: [w299 w304] -> w284
      tunnel: w285 -> [_ w302]
      tunnel: [w295 w300] -> w283
      tunnel: w286 -> [_ w303]
      frame False {
        n121 = Tick Count (ms)() -> (millisecond timer value=w294:u32)
        n122 = call "Read tower Operation.vi"() -> ("Command Info"=w293:T20, "Command Timing"=w292:cluster{"Start Time (ms)":u32, "Iterations":i32})  [unwired: 9 in, 1 out]
        n123 = Unbundle(w292) -> ("Start Time (ms)"=w298:u32, "Iterations"=w296:i32)
        n124 = Unbundle(w293) -> ("Status"=w299:T1)  [unwired: 2 out]
        n125 = Subtract(x=w294, y=w298) -> (x-y=w297:u32)
        n126 = Bundle(w297, "Iterations"=w296) -> (w295:cluster{u32, "Iterations":i32})  [unwired: 1 in]
      }
      frame True {
        n127 = call "tower Command Helper.vi"("Description"=w303, "SubSystem Data"=w302) -> ("Command Info Out"=w301:T20, "Command Timing"=w300:cluster{"Start Time (ms)":u32, "Iterations":i32})  [unwired: 7 in, 1 out]
        n128 = Unbundle(w301) -> ("Status"=w304:T1)  [unwired: 2 out]
      }
    }
    "Status" <- w284
    "Command Timing" <- w283
    n129 = global read "tower Published Globals.vi" "TowerLastCommandStatus"() -> (→"TowerLastCommandStatus":T1)
    n130 = Wait (ms)(milliseconds to wait=u32 20) -> ()  [unwired: 1 out]
  }
